vi "Test_CoderAndAI.vi"() -> ()   [LabVIEW 2017]
doc: "Use this template to build a producer/consumer design pattern with events to produce queue items. Use this design pattern instead of the User Interface Event Handler pattern for user interfaces when you want to execute code asynchronously in response to an event without slowing the user interface responsiveness."
uses:
  Controls/SV_CoderAndAI.ctl
  Controls/FV_CI Encoder Position.ctl
  <vilib>/ErrorRing/Error Ring.xnode
panel:
  out "ActualRate":dbl
  in  "Update Rate":bool
  out "Acquired Data":dbl[](array[numeric])
  in  "Sample Rate":dbl
  in  "Start":bool
  in  "stop":bool
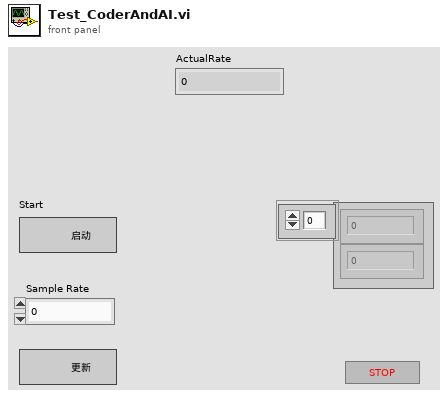
[diagram p1: front panel]
types:
  T1 = typedef "SV_CoderAndAI.ctl" = enum16{"Initialize", "Create Chennels", "Time Setting", "Start Daq", "Read Data", "CleanUp"}
  T2 = typedef "FV_CI Encoder Position.ctl" = enum16{"Channel Setting", "Timing Setting", "Trigger Setting", "Task Start", "Acquire Data", "Task Release"}
  T3 = cluster{"Counter":tag, "A Input Terminal":tag, "B Input Terminal":tag, "Pulses Per Revolution":u32, "Z Index Enable":bool, "Z Index Terminal":tag}
  T4 = cluster{"Sample Clock Source":tag, "Sample Rate":dbl, "Samples per Loop":i32}
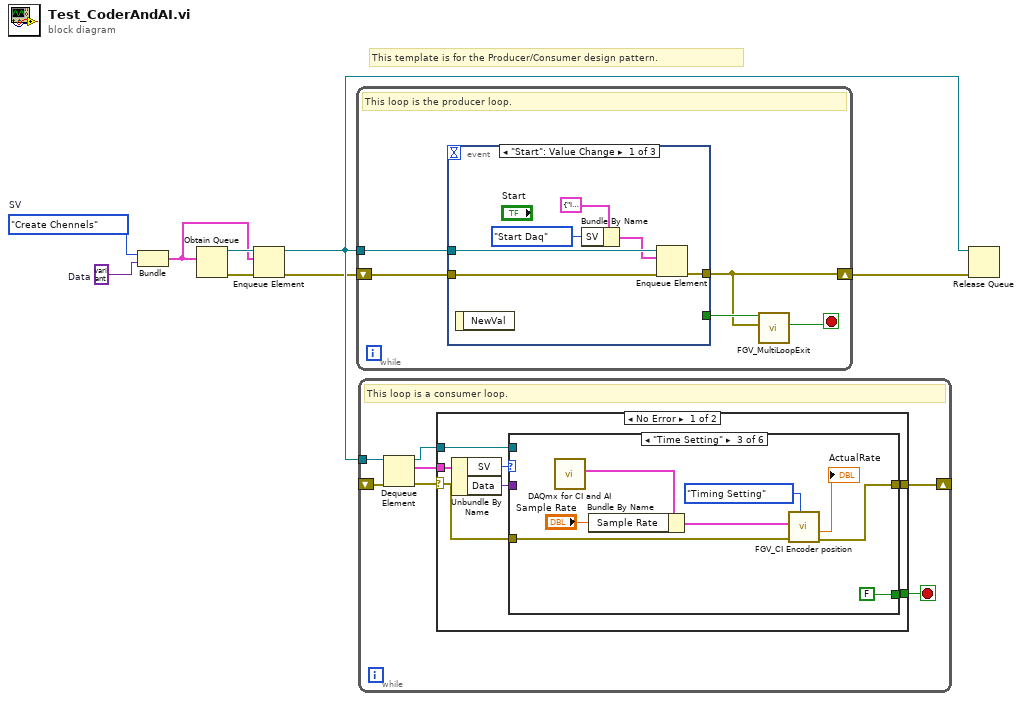
[diagram p0: block diagram]
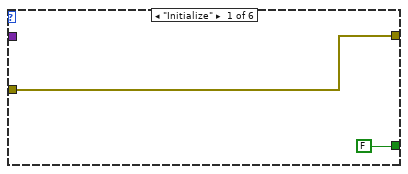
[diagram p2: hidden frame]
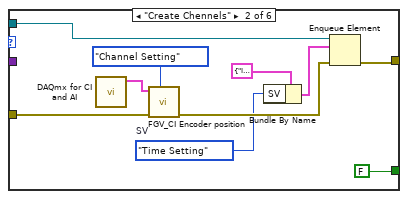
[diagram p3: hidden frame]
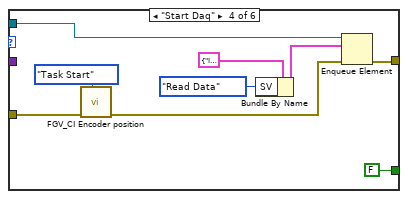
[diagram p4: hidden frame]
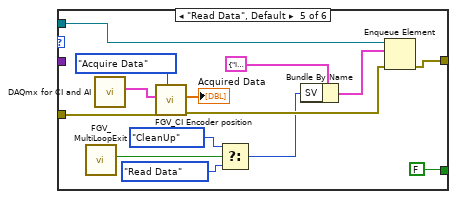
[diagram p5: hidden frame]
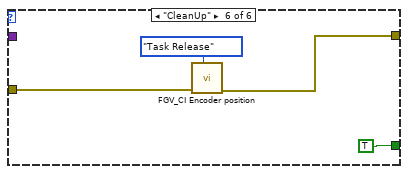
[diagram p6: hidden frame]
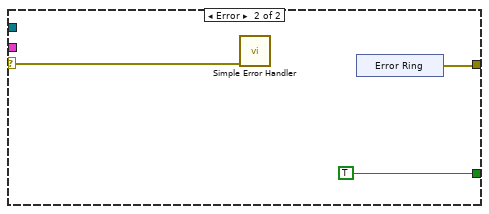
[diagram p7: hidden frame]
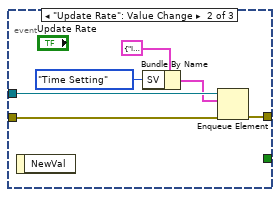
[diagram p8: hidden frame]
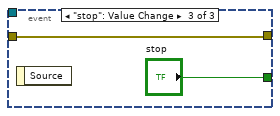
[diagram p9: hidden frame]
diagram:
  w5 = variant  # Data
  w6 = SV_CoderAndAI."Create Chennels"  # SV
  # "This template is for the Producer/Consumer design pattern."
  n1 = Bundle("SV"=w6, "Data"=w5) -> (w1:cluster{"SV":T1, "Data":variant})  [unwired: 1 in]
  n2 = Obtain Queue(element data type=w1) -> (queue out=w7:refnum<queue>, error out=w3:errorcluster)  [unwired: 4 in, 1 out]
  n3 = Enqueue Element(queue=w7, element=w1, error in (no error)=w3) -> (queue out=w4:refnum<queue>, error out=w2:errorcluster)  [unwired: 1 in, 1 out]
  n4 = while {
    shift-right: [w10] -> w8
    shift-left: w2 -> [w12]
    tunnel: w4 -> [w13]
    stop <- w9 stop-if-true
    # "This loop is the producer loop."
    n5 = event shown="[0] \"Start\": Value Change" {
      selector: _ -> [_ _ _]
      dyn-events: _ -> [_ _ _]
      timeout: _ -> [_ _ _]
      tunnel: w13 -> [w19 w25 _]
      tunnel: w12 -> [w18 w24 w26]
      tunnel: [w17 w23 w26] -> w10
      tunnel: [_ _ "stop"] -> w11
      event "Start": Value Change {
        n6 = event-data() -> ()  [unwired: 1 in, 1 out]
        n7 = Bundle By Name(cluster=cluster{"SV":T1, "Data":variant} {"SV"=enum."Initialize", "Data"=variant} ("element"), "SV"=SV_CoderAndAI."Start Daq") -> (w15:cluster{"SV":T1, "Data":variant})
        n8 = Enqueue Element(queue=w19, element=w15, error in (no error)=w18) -> (error out=w17:errorcluster)  [unwired: 1 in, 2 out]
      }
      event "Update Rate": Value Change {
        n9 = event-data() -> ()  [unwired: 1 in, 1 out]
        n10 = Bundle By Name(cluster=cluster{"SV":T1, "Data":variant} {"SV"=enum."Initialize", "Data"=variant} ("element"), "SV"=SV_CoderAndAI."Time Setting") -> (w21:cluster{"SV":T1, "Data":variant})
        n11 = Enqueue Element(queue=w25, element=w21, error in (no error)=w24) -> (error out=w23:errorcluster)  [unwired: 1 in, 2 out]
      }
      event "stop": Value Change {
        n12 = event-data() -> ()  [unwired: 1 in, 1 out]
      }
    }
    n13 = call "FGV_MultiLoopExit.vi"("error in (no error)"=w10, "Input"=w11) -> ("Output"=w9:bool)  [unwired: 9 in]
  }
  n14 = while {
    tunnel: w4 -> [w34]
    shift-right: [w29] -> _
    shift-left: _ -> [w28]
    stop <- w31 stop-if-true
    # "This loop is a consumer loop."
    n15 = Dequeue Element(queue=w34, error in (no error)=w28) -> (queue out=w30:refnum<queue>, element=w32:cluster{"SV":T1, "Data":variant}, error out=w33:errorcluster)  [unwired: 1 in, 1 out]
    n16 = case shown="No Error" w33 {
      selector: w33 -> [w39 w90]
      tunnel: w32 -> [w38 _]
      tunnel: [w36 TRUE] -> w31
      tunnel: w30 -> [w37 _]
      tunnel: [w35 w89] -> w29
      frame No Error {
        n17 = Unbundle By Name(w38) -> ("SV"=w41:T1, "Data"=w40:variant)
        n18 = case shown="\"Time Setting\"" w41 {
          tunnel: w40 -> [_ _ _ _ _ _]
          tunnel: w39 -> [w43 w53 w61 w70 w84 w87]
          tunnel: w37 -> [_ w48 _ w66 w80 _]
          tunnel: [FALSE FALSE FALSE FALSE FALSE TRUE] -> w36
          tunnel: [w43 w49 w57 w67 w72 w85] -> w35
          frame "Initialize" {
          }
          frame "Create Chennels" {
            w45 = SV_CoderAndAI."Time Setting"  # SV
            n19 = call "DAQmx for CI and AI.vi"() -> ("CI Channel Setting"=w52:T3)  [unwired: 10 in, 1 out]
            n20 = call "FGV_CI Encoder position.vi"("Function"=FV_CI_Encoder_Position."Channel Setting", "error in"=w53, "Channel Setting"=w52) -> ("error out"=w50:errorcluster)  [unwired: 6 in, 2 out]
            n21 = Bundle By Name(cluster=cluster{"SV":T1, "Data":variant} {"SV"=enum."Initialize", "Data"=variant}, "SV"=w45) -> (w46:cluster{"SV":T1, "Data":variant})
            n22 = Enqueue Element(queue=w48, element=w46, error in (no error)=w50) -> (error out=w49:errorcluster)  [unwired: 1 in, 2 out]
          }
          frame "Time Setting" {
            n23 = call "DAQmx for CI and AI.vi"() -> ("CI Timing Setting"=w59:T4)  [unwired: 10 in, 1 out]
            n24 = Bundle By Name(cluster=w59, "Sample Rate"="Sample Rate") -> (w58:T4)
            n25 = call "FGV_CI Encoder position.vi"("Function"=FV_CI_Encoder_Position."Timing Setting", "error in"=w61, "Timing Setting"=w58) -> ("error out"=w57:errorcluster, "ActualRate"=→"ActualRate":dbl)  [unwired: 6 in, 1 out]
          }
          frame "Start Daq" {
            n26 = call "FGV_CI Encoder position.vi"("Function"=FV_CI_Encoder_Position."Task Start", "error in"=w70) -> ("error out"=w68:errorcluster)  [unwired: 7 in, 2 out]
            n27 = Bundle By Name(cluster=cluster{"SV":T1, "Data":variant} {"SV"=enum."Initialize", "Data"=variant} ("element"), "SV"=SV_CoderAndAI."Read Data") -> (w64:cluster{"SV":T1, "Data":variant})
            n28 = Enqueue Element(queue=w66, element=w64, error in (no error)=w68) -> (error out=w67:errorcluster)  [unwired: 1 in, 2 out]
          }
          frame "Read Data", Default {
            n29 = call "FGV_MultiLoopExit.vi"() -> ("Output"=w79:bool)  [unwired: 11 in]
            n30 = call "DAQmx for CI and AI.vi"() -> ("CI Timing Setting"=w83:T4)  [unwired: 10 in, 1 out]
            n31 = call "FGV_CI Encoder position.vi"("Function"=FV_CI_Encoder_Position."Acquire Data", "error in"=w84, "Timing Setting"=w83) -> ("error out"=w81:errorcluster, "Acquired Data"=→"Acquired Data":dbl[])  [unwired: 6 in, 1 out]
            n32 = Select(t=SV_CoderAndAI."CleanUp" ("SV"), s=w79, f=SV_CoderAndAI."Read Data" ("SV")) -> (s? t:f=w74:T1)
            n33 = Bundle By Name(cluster=cluster{"SV":T1, "Data":variant} {"SV"=enum."Initialize", "Data"=variant}, "SV"=w74) -> (w75:cluster{"SV":T1, "Data":variant})
            n34 = Enqueue Element(queue=w80, element=w75, error in (no error)=w81) -> (error out=w72:errorcluster)  [unwired: 1 in, 2 out]
          }
          frame "CleanUp" {
            n35 = call "FGV_CI Encoder position.vi"("Function"=FV_CI_Encoder_Position."Task Release", "error in"=w87) -> ("error out"=w85:errorcluster)  [unwired: 7 in, 2 out]
          }
        }
      }
      frame Error {
        n36 = call <vilib>:"Simple Error Handler.vi"("error in (no error)"=w90) -> ()  [unwired: 4 in, 5 out]
        n37 = xnode "Error Ring"() -> ("error out"=w89:errorcluster)
      }
    }
  }
  n38 = Release Queue(queue=w4, error in (no error)=w8) -> ()  [unwired: 1 in, 3 out]
